vi "add new data to graph demo.vi"() -> ()   [LabVIEW 2013]
panel:
  out "Array":dbl[](array[numeric])
  in  "Stop":bool
  in  "# Plots":i32=2
  out "Graph":cluster{timestamp[], dbl[]}[](graph)
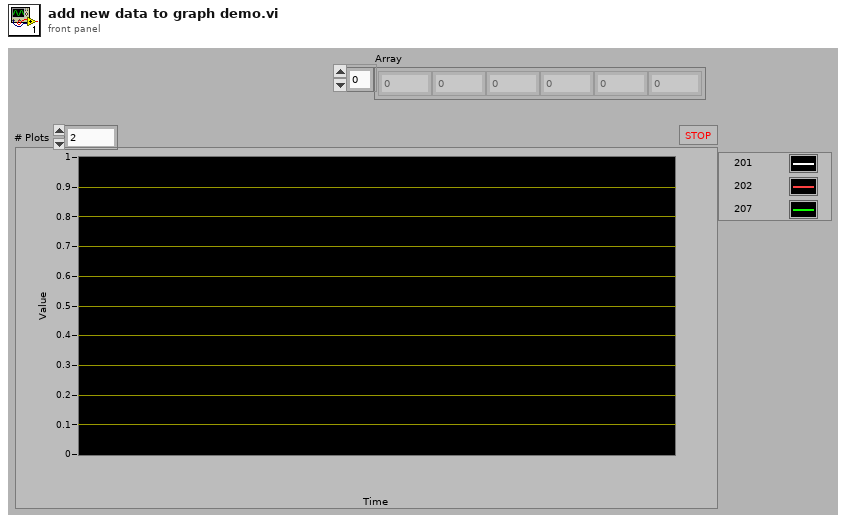
[diagram p1: front panel]
types:
  T1 = cluster{"Timestamp":timestamp[], "Data Array":dbl[]}[]
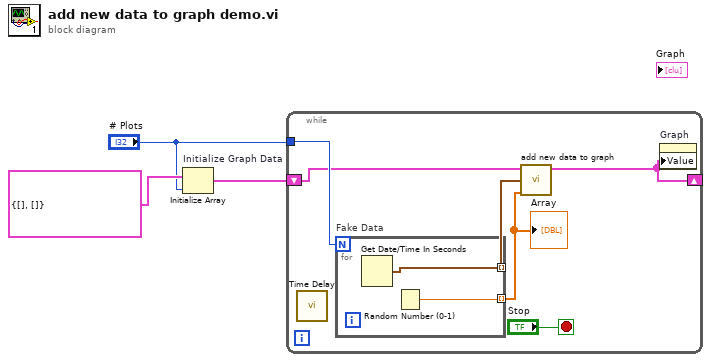
[diagram p0: block diagram]
diagram:
  n1 = Initialize Array "Initialize Graph Data"(cluster{timestamp[], dbl[]} {[], []} ("Graph i"), "# Plots") -> (w1:cluster{timestamp[], dbl[]}[])
  n2 = while {
    shift-right: [w4] -> _
    shift-left: w1 -> [w5]
    tunnel: "# Plots" -> [w8]
    stop <- "Stop" stop-if-true
    n3 = call "Time Delay"() -> ()  [unwired: 11 in, 1 out]
    n4 = for "Fake Data" {
      N: w8 -> [_]
      tunnel: [w11] -> w6 mode=indexing
      tunnel: [w10] -> w7 mode=indexing
      n5 = Get Date/Time In Seconds() -> (seconds since 1Jan1904=w10:timestamp)
      n6 = Random Number (0-1)() -> (number: 0 to 1=w11:dbl)
    }
    "Array" <- w6
    n7 = call "add new data to graph.vi"("New Timestamps"=w7, "Data Array"=w6, "Graph Data"=w5) -> ("Graph Data 2"=w4:T1)  [unwired: 7 in]
    n8 = property on="Graph" class="XYGraph (strict)"("Value"=w4) -> ()  [unwired: 2 in, 2 out]
  }
